vi "Tick Count with Error.vi"(7 "UsePrevious":bool=TRUE, 8 "error in (no error)":errorcluster, 11 "millisecond val in":u32) -> (0 "error out":errorcluster, 2 "Time":u32, 3 "millisecond timer value":u32)   [LabVIEW 2017]
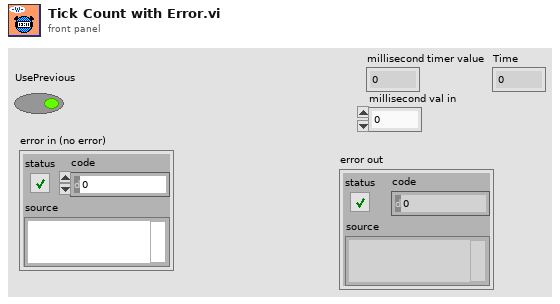
[diagram p1: front panel]
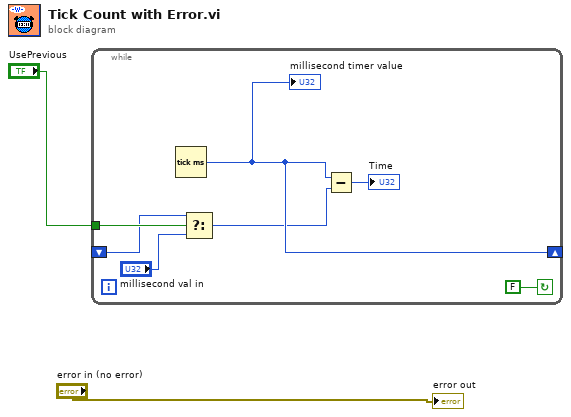
[diagram p0: block diagram]
diagram:
  n1 = while {
    shift-right: [w7] -> _
    shift-left: _ -> [w4]
    tunnel: "UsePrevious" -> [w6]
    stop <- FALSE continue-if-true
    n2 = Tick Count (ms)() -> (millisecond timer value=w7:u32)
    "millisecond timer value" <- w7
    n3 = Select(t=w4, s=w6, f="millisecond val in") -> (s? t:f=w3:u32)
    n4 = Subtract(x=w7, y=w3) -> (x-y=→"Time":u32)
  }
  "error out" <- "error in (no error)"
